vi "uA_daq_Initial_Aquire_mode.vi"(8 "error in":errorcluster, 10 "Acquire Mode":enum16{"Streaming", "Read All", "Stop"}(ring), 11 "USB DAQ":tag) -> (0 "error out":errorcluster, 3 "Refnum out":refnum<k21>)   [LabVIEW 2015]
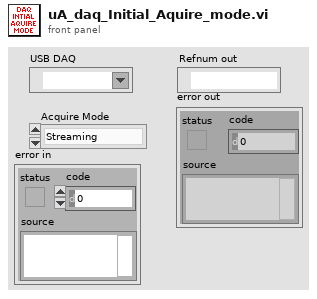
[diagram p1: front panel]
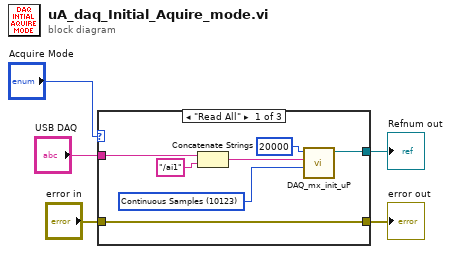
[diagram p0: block diagram]
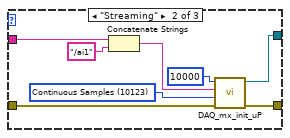
[diagram p2: hidden frame]
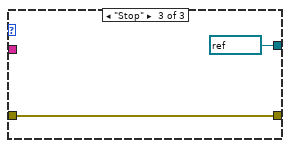
[diagram p3: hidden frame]
diagram:
  n1 = case shown="\"Read All\"" "Acquire Mode" {
    tunnel: [w8 w16 refnum<k21> "Stop" ("task out")] -> w4
    tunnel: "USB DAQ" -> [w7 w15 _]
    tunnel: "error in" -> [w6 w14 w21]
    tunnel: [w6 w13 w21] -> w1
    frame "Read All" {
      w10 = 10123 items=["Finite Samples"=10178, "Continuous Samples"=10123, "Hardware Timed Single Point"=12522] ("sample mode")
      n2 = Concatenate Strings(w7, "/ai1" ("string")) -> (w11:string)
      n3 = call "DAQ_mx_init_uP.vi"("sample mode"=w10, "physical channel"=w11, "number of samples"=20000 ("samples")) -> ("task out"=w8:refnum<k21>)  [unwired: 7 in, 1 out]
    }
    frame "Streaming" {
      w18 = 10123 items=["Finite Samples"=10178, "Continuous Samples"=10123, "Hardware Timed Single Point"=12522] ("sample mode")
      n4 = Concatenate Strings(w15, "/ai1" ("string")) -> (w19:string)
      n5 = call "DAQ_mx_init_uP.vi"("error in"=w14, "sample mode"=w18, "physical channel"=w19, "number of samples"=10000 ("samples")) -> ("error out"=w13:errorcluster, "task out"=w16:refnum<k21>)  [unwired: 6 in]
    }
    frame "Stop" {
    }
  }
  "Refnum out" <- w4
  "error out" <- w1
